vi "Transfer Setup Unified Control.vi"() -> ()   [LabVIEW 2014]
uses:
  BK9120/Serial_Config.ctl
  Omega/Serial_Config_Omega.ctl
  Meter_VI.ctl
  Omega/Omega CN9600 series.lvclass
  BK9120/B&K Precision 9120 series.lvclass
  <vilib>/Utility/error.llb/DialogType.ctl
  global/Global Variables.vi
panel:
  out "Omega":bool
  out "B&K":bool
  in  "Limit Value":dbl format="%#_4pA"
  in  "Ramp Control":bool
  in  "Operation to take (Limit Temp)":enum16{"Hold", "Turn off"}(ring) caption="Operation to take"
  in  "Temp. Limit":dbl min=0.0 max=200.0 step=1.0 format="%.1f"
  in  "Limit Temperature":bool
  in  "Operation to take (Limit Ramp)":enum16{"Hold", "Turn off"}(ring) caption="Operation to take"
  in  "Limit Variable":enum16{"Current", "Power", "Voltage"}(ring)
  in  "Limit Ramp":bool
  in  "Ramp Variable":enum16{"Current", "Power", "Voltage"}(ring)
  in  "Ramp Rate":dbl min=-50.0 max=50.0 step=0.0005 format="%#_3pA/min"
  out "Temperature Chart":dbl(graph)
  out "Omega Connected":bool caption="Connected"
  in  "Omega Con/Discon":bool
  in  "Omega Set Point":dbl caption="Set Point \n(internal temp. controller)" format="%.1f"
  out "Temperature":dbl format="%.1f"
  in  "Stop Button":bool
  in  "En/Disen Output":bool
  out "Operation Mode":u8(ring) items=["OFF", "Const. Curr", "Const. Volt"]
  out "Waveform Chart":cluster{"Current":dbl, "Voltage":dbl, dbl}(graph)
  out "Measured Impedence":dbl min=0.0 max=1.2 step=0.001 format="%_3p Ohm"
  in  "B&K UI Setpoint":T1 caption="Set Point" {"Current" min=0.0 max=1.2 step=0.001 format="%_5p A"; "Voltage" min=0.0 max=73.0 step=0.1 format="%_4p V"}
  out "Measured Power":dbl min=0.0 max=1.2 step=0.001 format="%_3p W"
  out "Measured":T1 {"Current" min=0.0 max=1.2 step=0.001 format="%_5p A"; "Voltage" min=0.0 max=73.0 step=0.1 format="%_4p V"}
  out "B&K Connected":bool caption="Connected"
  in  "BK Con/Discon":bool
  in  "Omega Connection":T2={"Baud"=9600, "Flow Ctl"=0, "Parity"=0, "COM Port"="COM2", "Address"=1} caption="Connection" {"Parity" items=["None", "Odd", "Even"]; "Flow Ctl" items=["None"]; "Baud" items=["4800"=4800, "9600"=9600, "19200"=19200, "38400"=38400]}
  in  "B&K Connection":T3={"Baud"=38400, "Flow Ctl"=0, "COM port"="COM1", "Parity"=0} caption="Connection" {"Parity" items=["None", "Odd", "Even"]; "Flow Ctl" items=["None"]; "Baud" items=["4800"=4800, "9600"=9600, "19200"=19200, "38400"=38400]}
  # "Omega CN96211 Temperature Controller"
  # "B&K Precision 9124 DC Power Supply"
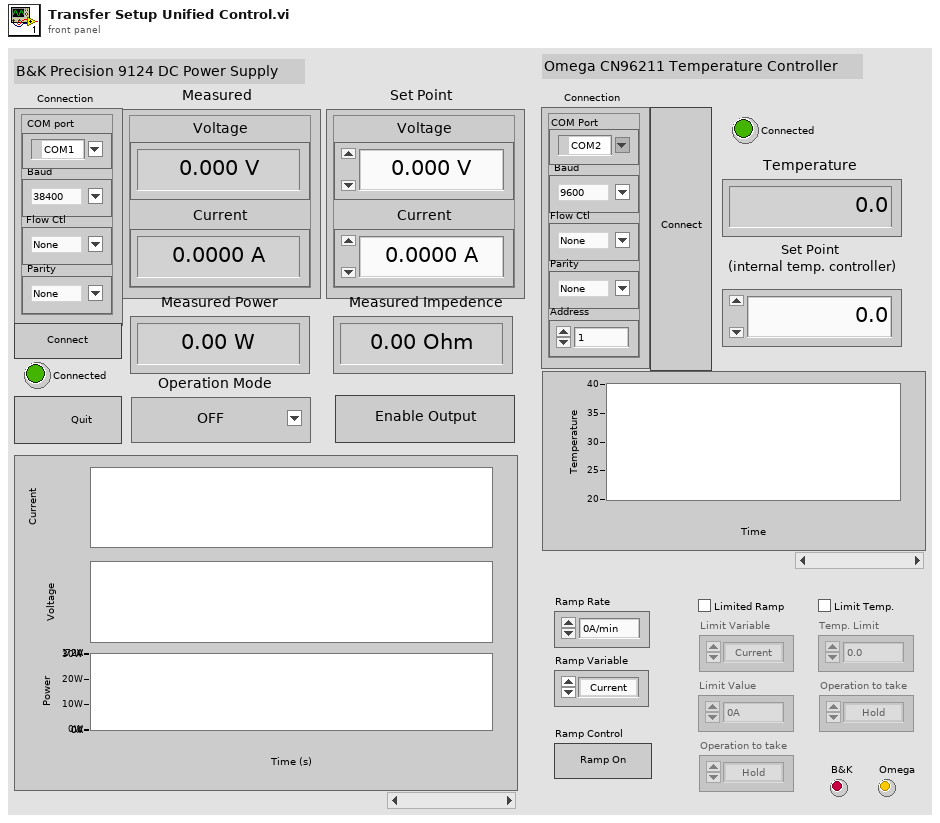
[diagram p1: front panel]
types:
  T1 = typedef "Meter_VI.ctl" = cluster{"Voltage":dbl, "Current":dbl}
  T2 = typedef "Omega CN9600 series.lvclass/Serial_Config_Omega.ctl" = cluster{"Baud":u32, "Flow Ctl":u16, "Parity":u16, "COM Port":refnum<visa-resource-name>, "Address":u8}
  T3 = typedef "B&K Precision 9120 series.lvclass/Serial_Config.ctl" = cluster{"Baud":u32, "Flow Ctl":u16, "COM port":refnum<visa-resource-name>, "Parity":u16}
  T4 = enum8{"Enabled", "Disabled", "Disabled and Grayed Out"}
  T5 = cluster{"Omega 96211":refnum<class "Omega CN9600 series.lvclass">, "B&K Precision":refnum<class "B&K Precision 9120 series.lvclass">, "B&K connected":bool, "Omega connected":bool, "Ramp On":bool, "Output Enabled":bool, "Limit temp":bool, "Limit ramp":bool, "B&K last update":u32, "Omega last update":u32, "Ramp Variable":enum16{"Current", "Power", "Voltage"}, "Limit Variable":enum16{"Current", "Power", "Voltage"}}
  T6 = enum32{"invalid app kind", "Development System", "Run Time System", "Student Edition", "Embedded LabVIEW", "Evaluation", "Custom"}
  T7 = typedef "DialogType.ctl" = u16
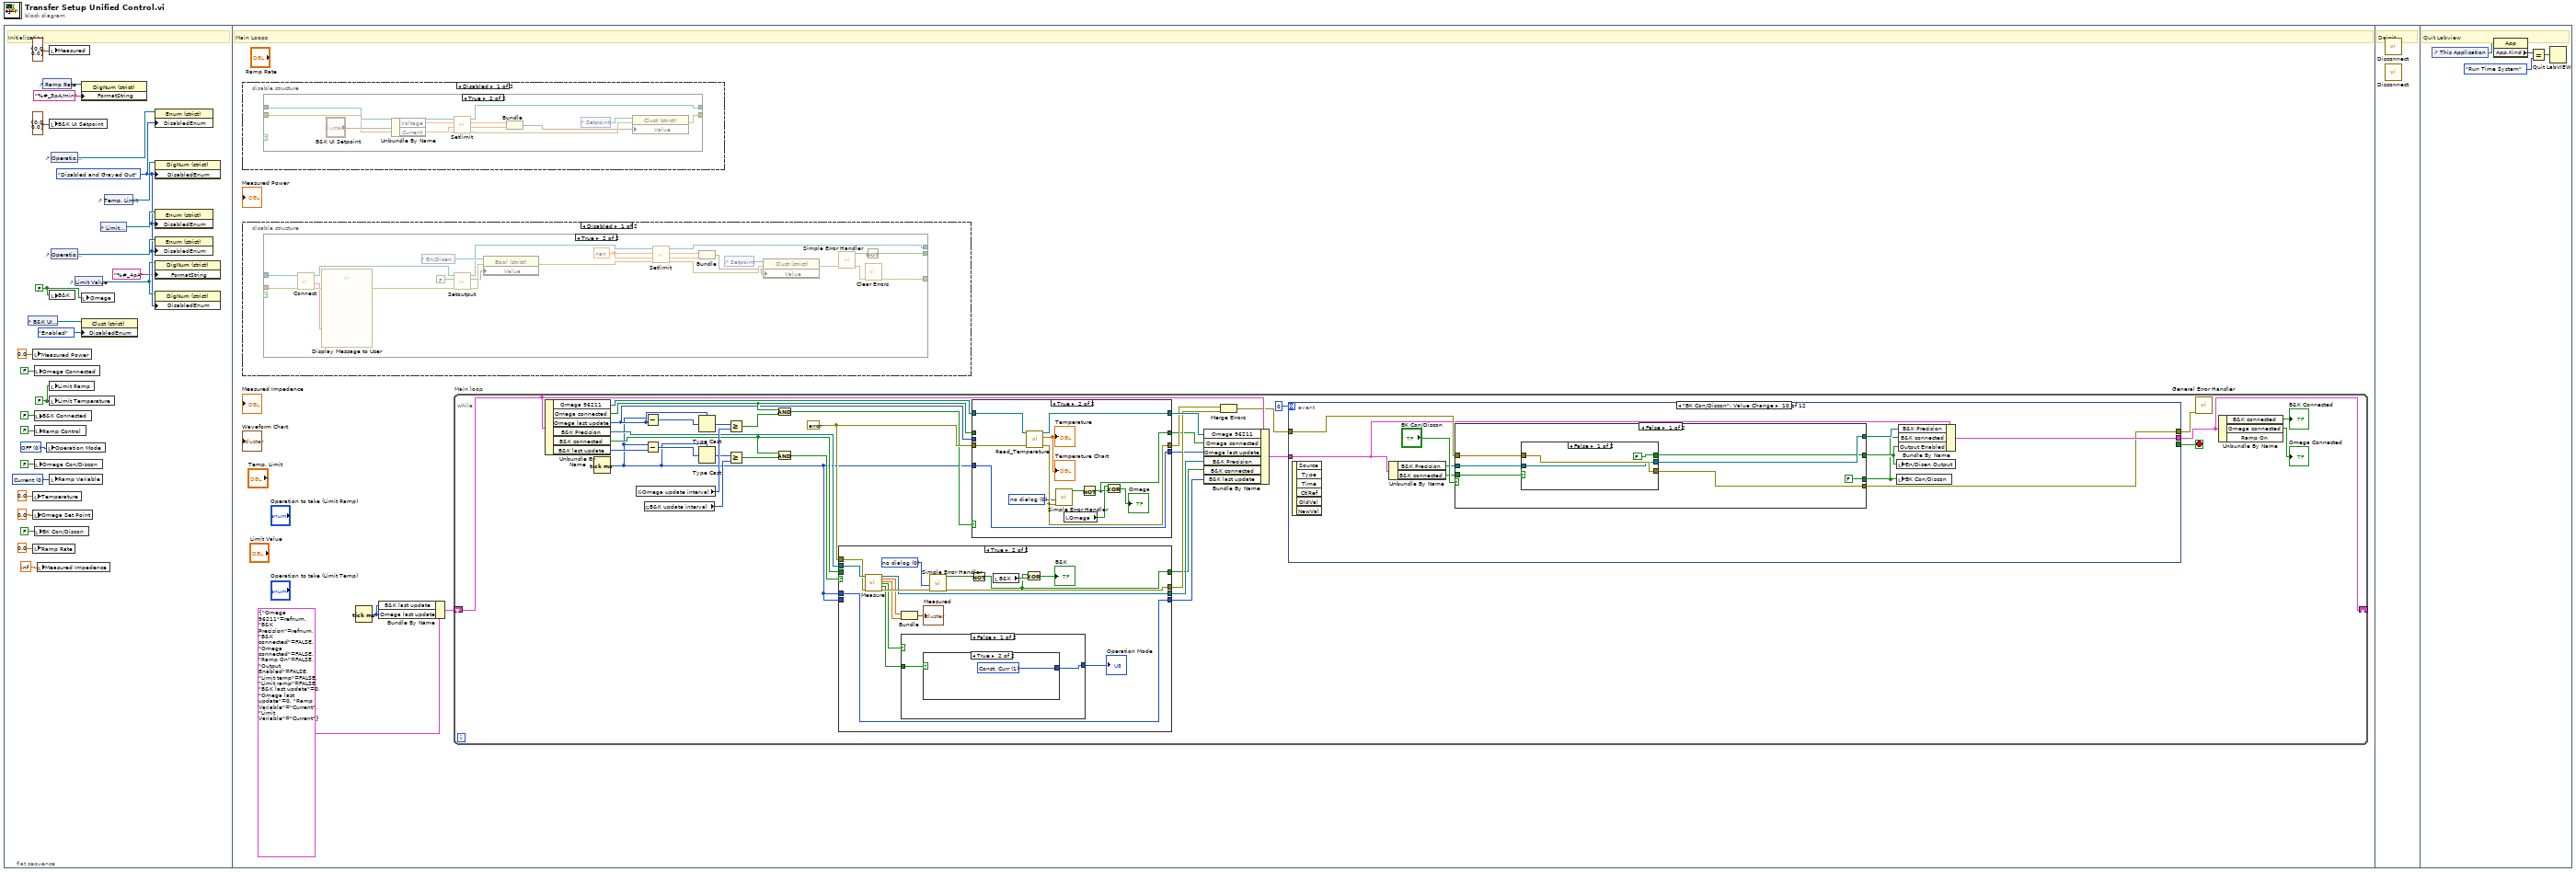
[diagram p0: block diagram]
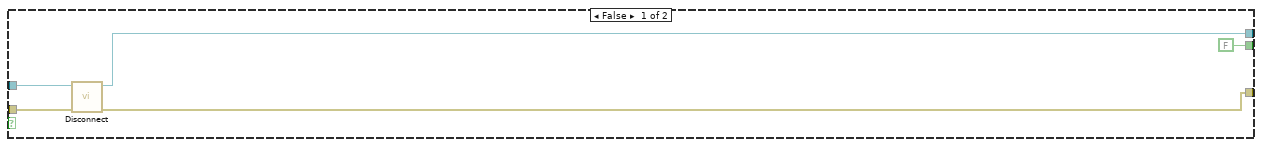
[diagram p4: hidden frame]
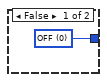
[diagram p7: hidden frame]
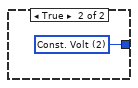
[diagram p8: hidden frame]
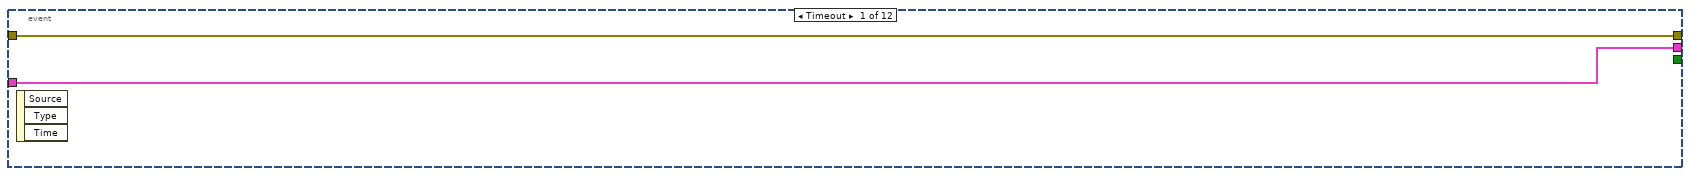
[diagram p10: hidden frame]
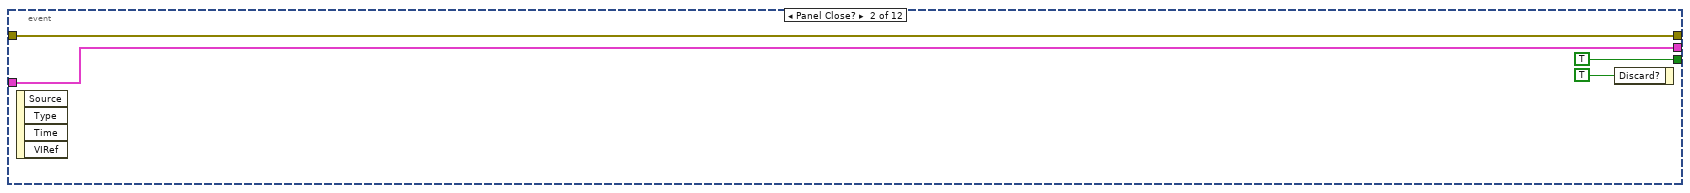
[diagram p11: hidden frame]
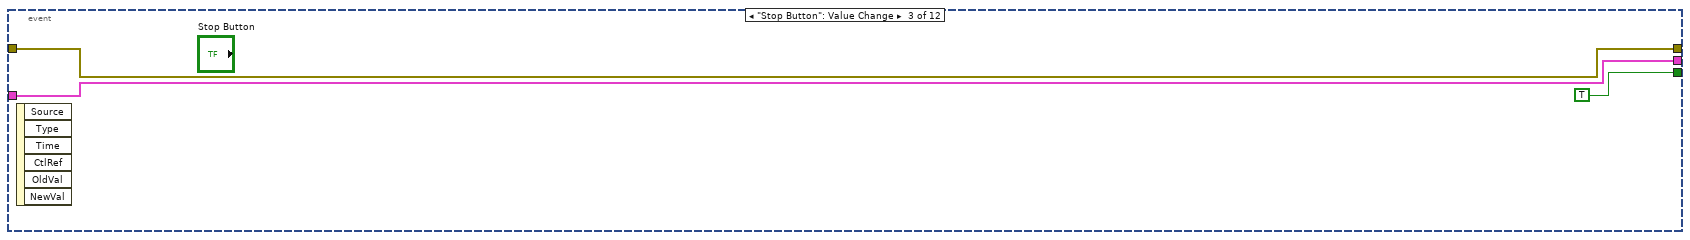
[diagram p12: hidden frame]
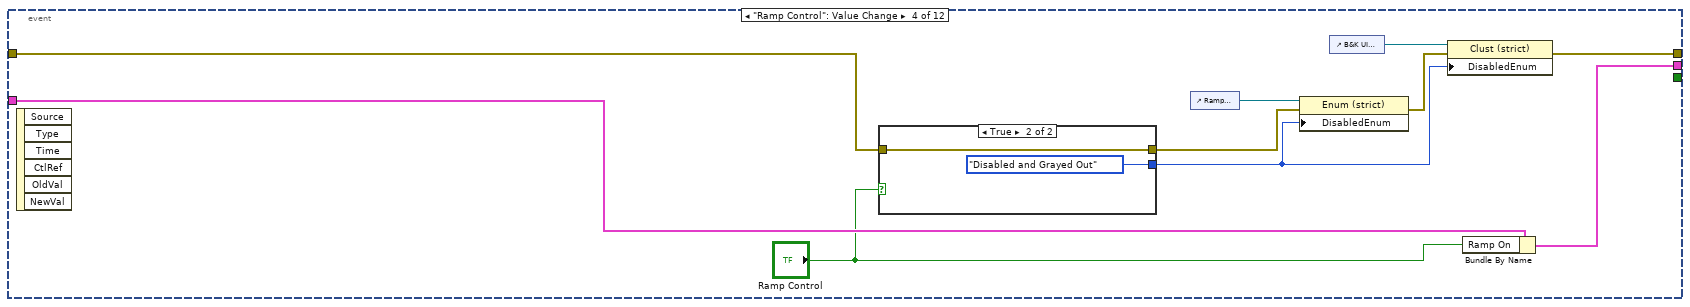
[diagram p13: hidden frame]
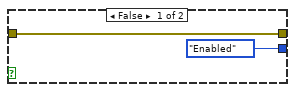
[diagram p14: hidden frame]
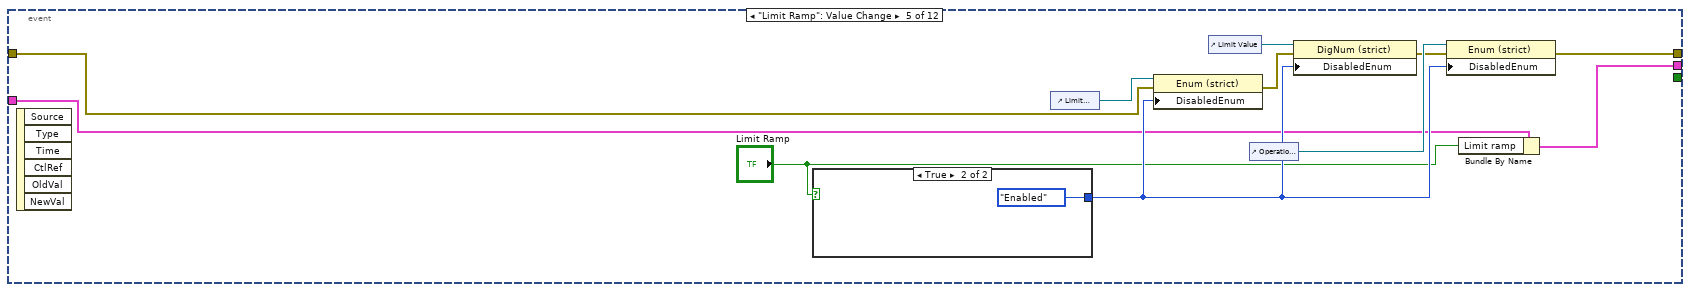
[diagram p15: hidden frame]
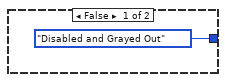
[diagram p16: hidden frame]
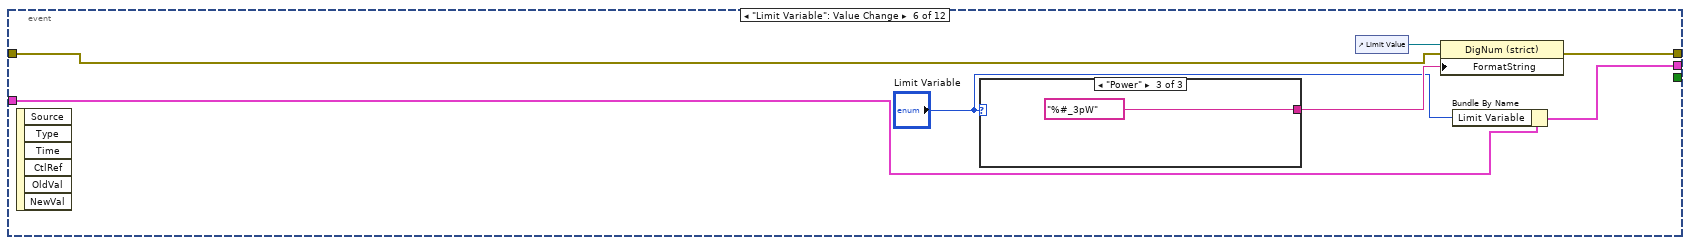
[diagram p17: hidden frame]
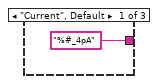
[diagram p18: hidden frame]
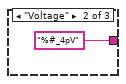
[diagram p19: hidden frame]
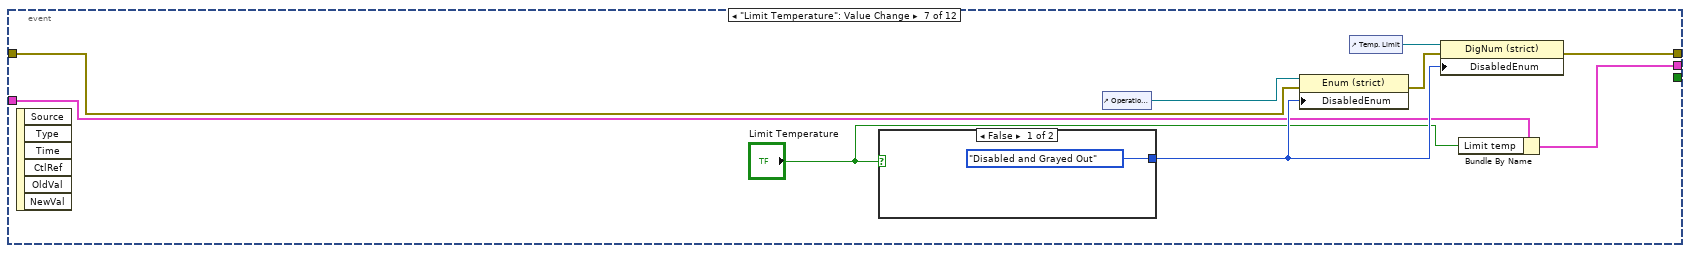
[diagram p20: hidden frame]
diagram:
  n1 = flat-sequence {
    frame #0 {
      w1 = FALSE
      w6 = T4."Disabled and Grayed Out" ("Disabled")
      w11 = FALSE ("Limit Ramp")
      w16 = u16 0 items=["Current", "Power", "Voltage"] ("Ramp Variable")
      w18 = u8 0 items=["OFF", "Const. Curr", "Const. Volt"] ("Operation Mode")
      # "Initialization"
      n2 = control-ref of="B&K UI Setpoint"() -> (w3:refnum<vi>)
      n3 = local write "Measured Power"(0.0 ("Measured Power")) -> ()
      n4 = local write "Temperature"(0.0 ("Temperature")) -> ()
      n5 = local write "Omega Set Point"(0.0 ("Omega Set Point")) -> ()
      n6 = local write "Ramp Rate"(0.0 ("Ramp Rate")) -> ()
      n7 = local write "Omega Connected"(FALSE ("Omega Connected")) -> ()
      n8 = local write "B&K Connected"(FALSE ("B&K Connected")) -> ()
      n9 = local write "Ramp Control"(FALSE ("Ramp Control")) -> ()
      n10 = local write "Omega Con/Discon"(FALSE ("Omega Con/Discon")) -> ()
      n11 = local write "BK Con/Discon"(FALSE ("BK Con/Discon")) -> ()
      n12 = local write "Measured Impedence"(inf ("Measured Impedence")) -> ()
      n13 = control-ref of="Ramp Rate"() -> (w9:refnum<vi>)
      n14 = local write "Operation Mode"(w18) -> ()
      n15 = local write "Measured"(T1 {"Voltage"=0.0, "Current"=0.0} ("Measured")) -> ()
      n16 = local write "B&K UI Setpoint"(T1 {"Voltage"=0.0, "Current"=0.0} ("Setpoint")) -> ()
      n17 = local write "B&K"(w1) -> ()
      n18 = local write "Limit Ramp"(w11) -> ()
      n19 = local write "Limit Temperature"(w11) -> ()
      n20 = local write "Ramp Variable"(w16) -> ()
      n21 = control-ref of="Operation to take (Limit Temp)"() -> (w13:refnum<vi>)
      n22 = control-ref of="Operation to take (Limit Ramp)"() -> (w14:refnum<vi>)
      n23 = control-ref of="Limit Value"() -> (w5:refnum<vi>)
      n24 = property class="DigNum (strict)"(reference=w9, "FormatString"="%#_3pA/min" ("Format String")) -> ()  [unwired: 1 in, 2 out]
      n25 = local write "Omega"(w1) -> ()
      n26 = property class="Clust (strict)"(reference=w3, "DisabledEnum"=T4."Enabled" ("Disabled")) -> ()  [unwired: 1 in, 2 out]
      n27 = control-ref of="Limit Variable"() -> (w15:refnum<vi>)
      n28 = control-ref of="Temp. Limit"() -> (w12:refnum<vi>)
      n29 = property class="Enum (strict)"(reference=w13, "DisabledEnum"=w6) -> ()  [unwired: 1 in, 2 out]
      n30 = property class="DigNum (strict)"(reference=w12, "DisabledEnum"=w6) -> ()  [unwired: 1 in, 2 out]
      n31 = property class="Enum (strict)"(reference=w15, "DisabledEnum"=w6) -> ()  [unwired: 1 in, 2 out]
      n32 = property class="Enum (strict)"(reference=w14, "DisabledEnum"=w6) -> ()  [unwired: 1 in, 2 out]
      n33 = property class="DigNum (strict)"(reference=w5, "FormatString"="%#_4pA" ("Format String")) -> ()  [unwired: 1 in, 2 out]
      n34 = property class="DigNum (strict)"(reference=w5, "DisabledEnum"=w6) -> ()  [unwired: 1 in, 2 out]
    }
    frame #1 {
      # "Main Loops"
      n35 = disable-structure shown="Disabled" {
        frame Disabled {
          n36 = case shown="True" {
            selector: _ -> [_ _]
            tunnel: _ -> [w32 w44]
            tunnel: _ -> [w31 w40]
            tunnel: [w32 w37] -> _
            tunnel: [w31 w34] -> _
            frame False {
            }
            frame True {
              n37 = Unbundle By Name("B&K UI Setpoint") -> ("Voltage"=w41:dbl, "Current"=w42:dbl)
              n38 = call "Setlimit.vi"("error in (no error)"=w40, "Current"=w42, "Voltage"=w41, "B&K Precision 9120 series in"=w44) -> ("error out"=w35:errorcluster, "Current read"=w38:dbl, "Voltage read"=w39:dbl, "B&K Precision 9120 series out"=w37:refnum<class "B&K Precision 9120 series.lvclass">)  [unwired: 4 in]
              n39 = Bundle("Voltage read"=w39, "Current read"=w38) -> (w33:cluster{"Voltage read":dbl, "Current read":dbl})  [unwired: 1 in]
              n40 = control-ref of="Setpoint"() -> (w36:refnum<vi>)
              n41 = property class="Clust (strict)"(reference=w36, error in=w35, "Value"=w33) -> (error out=w34:errorcluster)  [unwired: 1 out]
            }
          }
        }
        frame Enabled {
        }
      }
      n42 = disable-structure shown="Disabled" {
        frame Disabled {
          n43 = case shown="True" {
            selector: _ -> [_ _]
            tunnel: _ -> [w49 w74]
            tunnel: _ -> [w48 w73]
            tunnel: [w46 w58] -> _
            tunnel: [w47 w66] -> _
            tunnel: [FALSE w69] -> _
            frame False {
              n44 = call "Disconnect.vi"("error in (no error)"=w48, "B&K Precision 9120 series in"=w49) -> ("error out"=w47:errorcluster, "B&K Precision 9120 series out"=w46:refnum<class "B&K Precision 9120 series.lvclass">)  [unwired: 8 in]
            }
            frame True {
              w56 = nan ("Voltage")
              n45 = call "Connect.vi"("error in (no error)"=w73, "B&K Precision 9120 series in"=w74) -> ("error out"=w71:errorcluster, "result"=w70:string, "B&K Precision 9120 series out"=w65:refnum<class "B&K Precision 9120 series.lvclass">, "Serial Config"=w72:T3)  [unwired: 6 in]
              n46 = call "Display Message to User"("error in (no error)"=w71, "Message"=w70) -> ("error out"=w63:errorcluster)  [unwired: 8 in, 1 out]
              n47 = control-ref of="En/Disen Output"() -> (w62:refnum<vi>)
              n48 = call "Setoutput.vi"("error in (no error)"=w63, "enable"=FALSE, "B&K Precision 9120 series in"=w65) -> ("error out"=w61:errorcluster, "actual_state"=w60:bool, "B&K Precision 9120 series out"=w59:refnum<class "B&K Precision 9120 series.lvclass">)  [unwired: 6 in]
              n49 = property class="Bool (strict)"(reference=w62, error in=w61, "Value"=w60) -> (error out=w57:errorcluster)  [unwired: 1 out]
              n50 = call "Setlimit.vi"("error in (no error)"=w57, "Current"=w56, "Voltage"=w56, "B&K Precision 9120 series in"=w59) -> ("error out"=w52:errorcluster, "Current read"=w54:dbl, "Voltage read"=w55:dbl, "B&K Precision 9120 series out"=w58:refnum<class "B&K Precision 9120 series.lvclass">)  [unwired: 4 in]
              n51 = Bundle("Voltage read"=w55, "Current read"=w54) -> (w50:cluster{"Voltage read":dbl, "Current read":dbl})  [unwired: 1 in]
              n52 = control-ref of="Setpoint"() -> (w53:refnum<vi>)
              n53 = property class="Clust (strict)"(reference=w53, error in=w52, "Value"=w50) -> (error out=w51:errorcluster)  [unwired: 1 out]
              n54 = call <vilib>:"Simple Error Handler.vi"("error in (no error)"=w51) -> ("error?"=w68:bool, "error out"=w67:errorcluster)  [unwired: 4 in, 3 out]
              n55 = Not(x=w68) -> (.not. x?=w69:bool)
              n56 = call <vilib>:"Clear Errors.vi"("error in (no error)"=w67) -> ("error out"=w66:errorcluster)  [unwired: 5 in, 1 out]
            }
          }
        }
        frame Enabled {
        }
      }
      n57 = Tick Count (ms)() -> (millisecond timer value=w30:u32)
      n58 = Bundle By Name(cluster=T5 {"Omega 96211"=refnum, "B&K Precision"=refnum, "B&K connected"=FALSE, "Omega connected"=FALSE, "Ramp On"=FALSE, "Output Enabled"=FALSE, "Limit temp"=FALSE, "Limit ramp"=FALSE, "B&K last update"=0, "Omega last update"=0, "Ramp Variable"=enum."Current", "Limit Variable"=enum."Current"}, "B&K last update"=w30, "Omega last update"=w30) -> (w29:T5)
      n59 = while "Main loop" {
        shift-right: [w90] -> _
        shift-left: w29 -> [w104]
        stop <- w108 stop-if-true
        w100 = errorcluster {"status"=FALSE, "code"=0, "source"=""} ("error constant")
        n60 = Unbundle By Name(w104) -> ("Omega 96211"=w106:refnum<class "Omega CN9600 series.lvclass">, "Omega connected"=w93:bool, "Omega last update"=w86:u32, "B&K Precision"=w79:refnum<class "B&K Precision 9120 series.lvclass">, "B&K connected"=w77:bool, "B&K last update"=w87:u32)
        n61 = Tick Count (ms)() -> (millisecond timer value=w75:u32)
        n62 = global read "Global Variables.vi" "Omega update interval"() -> (w98:u32)
        n63 = global read "Global Variables.vi" "B&K update interval"() -> (w83:u32)
        n64 = Subtract(x=w75, y=w86) -> (x-y=w92:u32)
        n65 = Subtract(x=w75, y=w87) -> (x-y=w85:u32)
        n66 = Type Cast(type=w86, x=w92) -> (*(type *) &x=w91:u32)
        n67 = Type Cast(type=w75, x=w85) -> (*(type *) &x=w84:u32)
        n68 = Greater Or Equal?(x=w91, y=w98) -> (x >= y?=w96:bool)
        n69 = Greater Or Equal?(x=w84, y=w83) -> (x >= y?=w81:bool)
        n70 = And(x=w93, y=w96) -> (x .and. y?=w97:bool)
        n71 = And(x=w77, y=w81) -> (x .and. y?=w82:bool)
        n72 = case shown="True" w82 {
          tunnel: w100 -> [w113 w129]
          tunnel: [w113 w126] -> w101
          tunnel: [w112 w124] -> w80
          tunnel: w79 -> [w112 w130]
          tunnel: w75 -> [w111 _]
          tunnel: [w111 w117] -> w78
          tunnel: w77 -> [w110 _]
          tunnel: [w110 w114] -> w76
          tunnel: w75 -> [_ w117]
          frame False {
          }
          frame True {
            w127 = T7 0 items=["no dialog", "OK message", "continue or stop message", "OK message + warnings", "continue/stop + warnings"] ("type of dialog (OK msg:1)")
            n73 = call "Measure.vi"("B&K Precision 9120 series in"=w130, "error in (no error)"=w129) -> ("B&K Precision 9120 series out"=w124:refnum<class "B&K Precision 9120 series.lvclass">, "Voltage"=w123:dbl, "Current"=w122:dbl, "CV"=w120:bool, "CC"=w119:bool, "error out"=w128:errorcluster)  [unwired: 12 in]
            n74 = Bundle("Voltage"=w123, "Current"=w122) -> (→"Measured":cluster{"Voltage":dbl, "Current":dbl})  [unwired: 1 in]
            n75 = case shown="False" w120 {
              tunnel: w119 -> [w132 _]
              tunnel: [w131 w135] -> w118
              frame False {
                n76 = case shown="True" w132 {
                  tunnel: [w133 w134] -> w131
                  frame False {
                    w133 = u8 0 items=["OFF", "Const. Curr", "Const. Volt"] ("Operation Mode")
                  }
                  frame True {
                    w134 = u8 1 items=["OFF", "Const. Curr", "Const. Volt"] ("Operation Mode")
                  }
                }
              }
              frame True {
                w135 = u8 2 items=["OFF", "Const. Curr", "Const. Volt"] ("Operation Mode")
              }
            }
            "Operation Mode" <- w118
            n77 = call <vilib>:"Simple Error Handler.vi"("type of dialog (OK msg:1)"=w127, "error in (no error)"=w128) -> ("error?"=w125:bool, "error out"=w126:errorcluster)  [unwired: 3 in, 3 out]
            n78 = Not(x=w125) -> (.not. x?=w114:bool)
            n79 = local read "B&K"() -> (w115:bool)
            n80 = Exclusive Or(1:w115, 2:w114) -> (0:→"B&K":bool)
          }
        }
        n81 = case shown="True" w97 {
          tunnel: w100 -> [w139 w149]
          tunnel: [w139 w146] -> w102
          tunnel: w106 -> [w138 w150]
          tunnel: [w138 w148] -> w105
          tunnel: w75 -> [_ w142]
          tunnel: [w136 w142] -> w95
          tunnel: [w137 w141] -> w94
          tunnel: w93 -> [w137 _]
          tunnel: w86 -> [w136 _]
          frame False {
          }
          frame True {
            w140 = T7 0 items=["no dialog", "OK message", "continue or stop message", "OK message + warnings", "continue/stop + warnings"] ("type of dialog (OK msg:1)")
            n82 = call "Read_Temperature.vi"("error in (no error)"=w149, "Omega CN9600 series.lvclass"=w150) -> ("error out"=w146:errorcluster, "Temperature"=→"Temperature" →"Temperature Chart":dbl, "Omega CN9600 series.lvclass 2"=w148:refnum<class "Omega CN9600 series.lvclass">)  [unwired: 7 in]
            n83 = call <vilib>:"Simple Error Handler.vi"("type of dialog (OK msg:1)"=w140, "error in (no error)"=w146) -> ("error?"=w145:bool)  [unwired: 3 in, 4 out]
            n84 = local read "Omega"() -> (w143:bool)
            n85 = Not(x=w145) -> (.not. x?=w141:bool)
            n86 = Exclusive Or(1:w141, 2:w143) -> (0:→"Omega":bool)
          }
        }
        n87 = Bundle By Name(cluster=w104, "Omega 96211"=w105, "Omega connected"=w94, "Omega last update"=w95, "B&K Precision"=w80, "B&K connected"=w76, "B&K last update"=w78) -> (w103:T5)
        n88 = Merge Errors(w102, w101) -> (w99:errorcluster)
        n89 = event shown="[9] \"BK Con/Discon\": Value Change" {
          selector: _ -> [_ _ _ _ _ _ _ _ _ _ _ _]
          dyn-events: _ -> [_ _ _ _ _ _ _ _ _ _ _ _]
          timeout: 0 -> [_ _ _ _ _ _ _ _ _ _ _ _]
          tunnel: [_ TRUE TRUE _ _ _ _ _ _ _ _ _] -> w108
          tunnel: w99 -> [w151 w154 w158 w166 w177 w191 w199 w212 w224 w247 w294 w312]
          tunnel: [w151 w154 w158 w163 w174 w190 w197 w211 w221 w245 w291 w311] -> w107
          tunnel: w103 -> [w152 w153 w157 w162 w179 w189 w202 w210 w223 w246 w298 w316]
          tunnel: [w152 w153 w157 w161 w178 w188 w200 w208 w222 w249 w290 w315] -> w90
          event Timeout {
            n90 = event-data() -> ()  [unwired: 1 in, 3 out]
          }
          event Panel Close? {
            n91 = event-data() -> ()  [unwired: 1 in, 4 out]
            n92 = event-data("Discard?"=TRUE) -> ()  [unwired: 1 in, 1 out]
          }
          event "Stop Button": Value Change {
            n93 = event-data() -> ()  [unwired: 1 in, 6 out]
          }
          event "Ramp Control": Value Change {
            n94 = event-data() -> ()  [unwired: 1 in, 6 out]
            n95 = case shown="True" "Ramp Control" {
              tunnel: [T4."Enabled" ("Disabled") T4."Disabled and Grayed Out" ("Disabled")] -> w167
              tunnel: w166 -> [w170 w172]
              tunnel: [w170 w172] -> w165
              frame False {
              }
              frame True {
              }
            }
            n96 = control-ref of="Ramp Variable"() -> (w168:refnum<vi>)
            n97 = property class="Enum (strict)"(reference=w168, error in=w165, "DisabledEnum"=w167) -> (error out=w164:errorcluster)  [unwired: 1 out]
            n98 = control-ref of="B&K UI Setpoint"() -> (w169:refnum<vi>)
            n99 = property class="Clust (strict)"(reference=w169, error in=w164, "DisabledEnum"=w167) -> (error out=w163:errorcluster)  [unwired: 1 out]
            n100 = Bundle By Name(cluster=w162, "Ramp On"="Ramp Control") -> (w161:T5)
          }
          event "Limit Ramp": Value Change {
            n101 = event-data() -> ()  [unwired: 1 in, 6 out]
            n102 = case shown="True" "Limit Ramp" {
              tunnel: [T4."Disabled and Grayed Out" ("Disabled") T4."Enabled" ("Disabled")] -> w181
              frame False {
              }
              frame True {
              }
            }
            n103 = control-ref of="Limit Variable"() -> (w184:refnum<vi>)
            n104 = property class="Enum (strict)"(reference=w184, error in=w177, "DisabledEnum"=w181) -> (error out=w176:errorcluster)  [unwired: 1 out]
            n105 = control-ref of="Limit Value"() -> (w182:refnum<vi>)
            n106 = control-ref of="Operation to take (Limit Ramp)"() -> (w183:refnum<vi>)
            n107 = property class="DigNum (strict)"(reference=w182, error in=w176, "DisabledEnum"=w181) -> (error out=w175:errorcluster)  [unwired: 1 out]
            n108 = property class="Enum (strict)"(reference=w183, error in=w175, "DisabledEnum"=w181) -> (error out=w174:errorcluster)  [unwired: 1 out]
            n109 = Bundle By Name(cluster=w179, "Limit ramp"="Limit Ramp") -> (w178:T5)
          }
          event "Limit Variable": Value Change {
            n110 = event-data() -> ()  [unwired: 1 in, 6 out]
            n111 = case shown="\"Power\"" "Limit Variable" {
              tunnel: ["%#_4pA" ("Format String") "%#_4pV" ("Format String") "%#_3pW" ("Format String")] -> w192
              frame "Current", Default {
              }
              frame "Voltage" {
              }
              frame "Power" {
              }
            }
            n112 = control-ref of="Limit Value"() -> (w193:refnum<vi>)
            n113 = property class="DigNum (strict)"(reference=w193, error in=w191, "FormatString"=w192) -> (error out=w190:errorcluster)  [unwired: 1 out]
            n114 = Bundle By Name(cluster=w189, "Limit Variable"="Limit Variable") -> (w188:T5)
          }
          event "Limit Temperature": Value Change {
            n115 = event-data() -> ()  [unwired: 1 in, 6 out]
            n116 = case shown="False" "Limit Temperature" {
              tunnel: [T4."Disabled and Grayed Out" ("Disabled") T4."Enabled" ("Disabled")] -> w203
              frame False {
              }
              frame True {
              }
            }
            n117 = control-ref of="Operation to take (Limit Temp)"() -> (w205:refnum<vi>)
            n118 = property class="Enum (strict)"(reference=w205, error in=w199, "DisabledEnum"=w203) -> (error out=w198:errorcluster)  [unwired: 1 out]
            n119 = control-ref of="Temp. Limit"() -> (w204:refnum<vi>)
            n120 = property class="DigNum (strict)"(reference=w204, error in=w198, "DisabledEnum"=w203) -> (error out=w197:errorcluster)  [unwired: 1 out]
            n121 = Bundle By Name(cluster=w202, "Limit temp"="Limit Temperature") -> (w200:T5)
          }
          event "Ramp Variable": Value Change {
            n122 = event-data() -> ()  [unwired: 1 in, 6 out]
            n123 = case shown="\"Voltage\"" "Ramp Variable" {
              tunnel: ["%#_3pA/min" ("Format String") "%#_3pV/min" ("Format String") "%#_3pW/min" ("Format String")] -> w213
              frame "Current", Default {
              }
              frame "Voltage" {
              }
              frame "Power" {
              }
            }
            n124 = control-ref of="Ramp Rate"() -> (w214:refnum<vi>)
            n125 = property class="DigNum (strict)"(reference=w214, error in=w212, "FormatString"=w213) -> (error out=w211:errorcluster)  [unwired: 1 out]
            n126 = Bundle By Name(cluster=w210, "Ramp Variable"="Ramp Variable") -> (w208:T5)
          }
          event "Omega Con/Discon": Value Change {
            n127 = event-data() -> ()  [unwired: 1 in, 6 out]
            n128 = Unbundle By Name(w223) -> ("Omega 96211"=w225:refnum<class "Omega CN9600 series.lvclass">)
            n129 = case shown="True" "Omega Con/Discon" {
              tunnel: w225 -> [w227 w241]
              tunnel: w224 -> [w226 w239]
              tunnel: [w228 w236] -> w221
              tunnel: [FALSE w235] -> w218
              tunnel: [w227 w232] -> w220
              frame False {
                n130 = call "Disconnect.vi"("error in (no error)"=w226, "Omega CN9600 series.lvclass"=w227) -> ("error out"=w228:errorcluster)  [unwired: 9 in]
              }
              frame True {
                w237 = T7 0 items=["no dialog", "OK message", "continue or stop message", "OK message + warnings", "continue/stop + warnings"] ("type of dialog (OK msg:1)")
                n131 = call "Connect.vi"("error in (no error)"=w239, "Serial Config"="Omega Connection", "Omega CN9600 series.lvclass"=w241) -> ("error out"=w238:errorcluster, "Omega CN9600 series.lvclass 2"=w233:refnum<class "Omega CN9600 series.lvclass">)  [unwired: 7 in]
                n132 = call "Set_Read_Temperature_SP.vi"("error in (no error)"=w238, "setpoint"=nan, "Omega CN9600 series.lvclass"=w233) -> ("error out"=w236:errorcluster, "actual setpoint"=w230:dbl, "Omega CN9600 series.lvclass 2"=w232:refnum<class "Omega CN9600 series.lvclass">)  [unwired: 5 in]
                n133 = local write "Omega Set Point"(w230) -> ()
                n134 = call <vilib>:"Simple Error Handler.vi"("type of dialog (OK msg:1)"=w237, "error in (no error)"=w236) -> ("error?"=w234:bool)  [unwired: 3 in, 4 out]
                n135 = Not(x=w234) -> (.not. x?=w235:bool)
              }
            }
            n136 = Bundle By Name(cluster=w223, "Omega 96211"=w220, "Omega connected"=w218) -> (w222:T5)
            n137 = local write "Omega Con/Discon"(w218) -> ()
          }
          event "BK Con/Discon": Value Change {
            n138 = event-data() -> ()  [unwired: 1 in, 6 out]
            n139 = Unbundle By Name(w246) -> ("B&K Precision"=w250:refnum<class "B&K Precision 9120 series.lvclass">, "B&K connected"=w242:bool)
            n140 = case shown="False" "BK Con/Discon" {
              tunnel: w250 -> [w255 w288]
              tunnel: [w257 w272] -> w248
              tunnel: w247 -> [w254 w286]
              tunnel: [w256 w281] -> w245
              tunnel: [FALSE w279] -> w243
              tunnel: [w253 w270] -> w244
              tunnel: w242 -> [w252 _]
              frame False {
                n141 = case shown="False" w252 {
                  tunnel: [w260 w269] -> w257
                  tunnel: [w261 w268] -> w256
                  tunnel: w255 -> [w260 w267]
                  tunnel: w254 -> [w261 w265]
                  tunnel: [FALSE ("actual_state") w262] -> w253
                  frame False {
                  }
                  frame True {
                    n142 = call "Setoutput.vi"("error in (no error)"=w265, "enable"=FALSE, "B&K Precision 9120 series in"=w267) -> ("error out"=w264:errorcluster, "actual_state"=w262:bool, "B&K Precision 9120 series out"=w266:refnum<class "B&K Precision 9120 series.lvclass">)  [unwired: 6 in]
                    n143 = call "Disconnect.vi"("error in (no error)"=w264, "B&K Precision 9120 series in"=w266) -> ("error out"=w268:errorcluster, "B&K Precision 9120 series out"=w269:refnum<class "B&K Precision 9120 series.lvclass">)  [unwired: 8 in]
                  }
                }
              }
              frame True {
                w282 = T7 0 items=["no dialog", "OK message", "continue or stop message", "OK message + warnings", "continue/stop + warnings"] ("type of dialog (OK msg:1)")
                w284 = nan ("Voltage")
                n144 = call "Connect.vi"("error in (no error)"=w286, "Serial Config"="B&K Connection", "B&K Precision 9120 series in"=w288) -> ("error out"=w283:errorcluster, "B&K Precision 9120 series out"=w285:refnum<class "B&K Precision 9120 series.lvclass">)  [unwired: 6 in, 1 out]
                n145 = call "Setlimit.vi"("error in (no error)"=w283, "Current"=w284, "Voltage"=w284, "B&K Precision 9120 series in"=w285) -> ("error out"=w275:errorcluster, "Current read"=w277:dbl, "Voltage read"=w278:dbl, "B&K Precision 9120 series out"=w273:refnum<class "B&K Precision 9120 series.lvclass">)  [unwired: 4 in]
                n146 = Bundle("Voltage read"=w278, "Current read"=w277) -> (w276:cluster{"Voltage read":dbl, "Current read":dbl})  [unwired: 1 in]
                n147 = local write "B&K UI Setpoint"(w276) -> ()
                n148 = call "Setoutput.vi"("error in (no error)"=w275, "enable"=FALSE, "B&K Precision 9120 series in"=w273) -> ("error out"=w274:errorcluster, "actual_state"=w270:bool, "B&K Precision 9120 series out"=w272:refnum<class "B&K Precision 9120 series.lvclass">)  [unwired: 6 in]
                n149 = call <vilib>:"Simple Error Handler.vi"("type of dialog (OK msg:1)"=w282, "error in (no error)"=w274) -> ("error?"=w280:bool, "error out"=w281:errorcluster)  [unwired: 3 in, 3 out]
                n150 = Not(x=w280) -> (.not. x?=w279:bool)
              }
            }
            n151 = local write "En/Disen Output"(w244) -> ()
            n152 = local write "BK Con/Discon"(w243) -> ()
            n153 = Bundle By Name(cluster=w246, "B&K Precision"=w248, "B&K connected"=w243, "Output Enabled"=w244) -> (w249:T5)
          }
          event "En/Disen Output": Value Change {
            n154 = event-data() -> ()  [unwired: 1 in, 6 out]
            n155 = Unbundle By Name(w298) -> ("B&K Precision"=w296:refnum<class "B&K Precision 9120 series.lvclass">, "B&K connected"=w300:bool, "Output Enabled"=w289:bool)
            n156 = Exclusive Or(1:w289, 2:"En/Disen Output") -> (0:w299:bool)
            n157 = And(x=w300, y=w299) -> (x .and. y?=w297:bool)
            n158 = case shown="True" w297 {
              tunnel: w296 -> [w303 w309]
              tunnel: "En/Disen Output" -> [_ w308]
              tunnel: w294 -> [w301 w307]
              tunnel: [w302 w306] -> w293
              tunnel: [w303 w305] -> w292
              tunnel: [w301 w304] -> w291
              tunnel: w289 -> [w302 _]
              frame False {
              }
              frame True {
                n159 = call "Setoutput.vi"("error in (no error)"=w307, "enable"=w308, "B&K Precision 9120 series in"=w309) -> ("error out"=w304:errorcluster, "actual_state"=w306:bool, "B&K Precision 9120 series out"=w305:refnum<class "B&K Precision 9120 series.lvclass">)  [unwired: 6 in]
              }
            }
            n160 = Bundle By Name(cluster=w298, "B&K Precision"=w292, "Output Enabled"=w293) -> (w290:T5)
            n161 = local write "En/Disen Output"(w293) -> ()
          }
          event "Omega Set Point": Value Change {
            n162 = event-data() -> ()  [unwired: 1 in, 6 out]
            n163 = Unbundle By Name(w316) -> ("Omega 96211"=w317:refnum<class "Omega CN9600 series.lvclass">)
            n164 = call "Set_Read_Temperature_SP.vi"("error in (no error)"=w312, "setpoint"="Omega Set Point", "Omega CN9600 series.lvclass"=w317) -> ("error out"=w311:errorcluster, "actual setpoint"=w310:dbl, "Omega CN9600 series.lvclass 2"=w314:refnum<class "Omega CN9600 series.lvclass">)  [unwired: 5 in]
            n165 = local write "Omega Set Point"(w310) -> ()
            n166 = Bundle By Name(cluster=w316, "Omega 96211"=w314) -> (w315:T5)
          }
        }
        n167 = call <vilib>:"General Error Handler.vi"("error in (no error)"=w107) -> ()  [unwired: 10 in, 5 out]
        n168 = Unbundle By Name(w90) -> ("B&K connected"=→"B&K Connected":bool, "Omega connected"=→"Omega Connected":bool)  [unwired: 1 out]
      }
    }
    frame #2 {
      # "Deinit"
      n169 = call "Disconnect.vi"() -> ()  [unwired: 11 in, 1 out]
      n170 = call "Disconnect.vi"() -> ()  [unwired: 10 in, 2 out]
    }
    frame #3 {
      # "Quit Labview"
      n171 = control-ref of="This Application"() -> (w321:refnum<vi>)
      n172 = property class="App"(reference=w321) -> ("App.Kind"=w320:T6)  [unwired: 1 in, 2 out]
      n173 = Equal?(x=w320, y=T6."Run Time System") -> (x = y?=w318:bool)
      n174 = Quit LabVIEW(quit? (T)=w318) -> ()
    }
  }
